vi "RLC_close.vi"(11 "Path":path=path "H:/CDH/CDH_control/python_CDH") -> (3 "String":string)   [LabVIEW 2011]
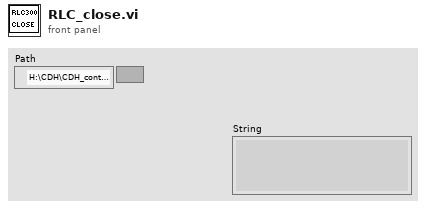
[diagram p1: front panel]
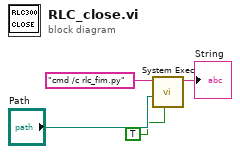
[diagram p0: block diagram]
diagram:
  n1 = call <vilib>:"System Exec.vi"("run minimized? (F)"=TRUE, "working directory"="Path", "command line"="cmd /c rlc_fim.py" ("String 2")) -> ("standard output"=→"String":string)  [unwired: 5 in, 3 out]
